vi "Write CFG File.vi"(7 "Section":string, 8 "error in (no error)":errorcluster, 10 "File refnum":T1, 11 "Mag Lab Parameters in":refnum<class "Mag Lab Parameters.lvclass">) -> (0 "error out":errorcluster, 2 "File refnum out":T1, 3 "Mag Lab Parameters out":refnum<class "Mag Lab Parameters.lvclass">)   [LabVIEW 2015, in "Mag Lab Parameters.lvclass"]
uses:
  Mag Lab Parameters.lvclass
  <vilib>/Utility/config.llb/Config Data RefNum.ctl
  <vilib>/Utility/config.llb/NI_LVConfig.lvlib
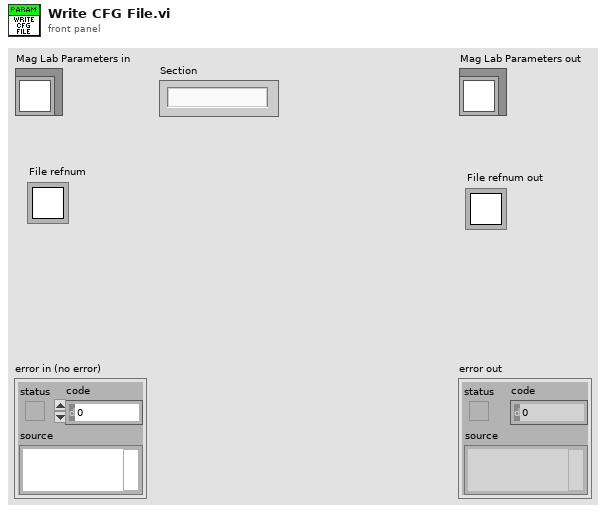
[diagram p1: front panel]
types:
  T1 = typedef "NI_LVConfig.lvlib/Config Data RefNum.ctl" = refnum<k1>
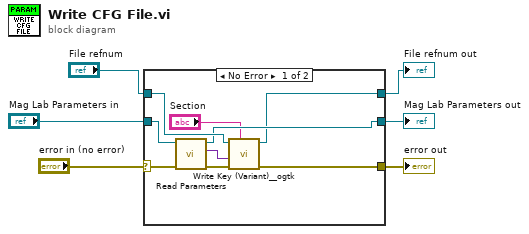
[diagram p0: block diagram]
diagram:
  n1 = case shown="No Error" "error in (no error)" {
    selector: "error in (no error)" -> [w8 w18]
    tunnel: [w9 w18] -> w5
    tunnel: [w13 w17] -> w3
    tunnel: "Mag Lab Parameters in" -> [w15 w17]
    tunnel: "File refnum" -> [w14 w16]
    tunnel: [w10 w16] -> w1
    frame No Error {
      n2 = call-dynamic "Read Parameters.vi"("error in (no error)"=w8, "Mag Lab Parameters in"=w15) -> ("error out"=w7:errorcluster, "Parameters"=w12:variant, "Mag Lab Parameters out"=w13:refnum<class "Mag Lab Parameters.lvclass">)  [unwired: 7 in]
      n3 = call <userlib>:"Write Key (Variant)__ogtk.vi"("section"="Section", "error in (no error)"=w7, "key-value"=w12, "refnum"=w14) -> ("error out"=w9:errorcluster, "refnum out"=w10:T1)  [unwired: 6 in]
    }
    frame Error {
    }
  }
  "error out" <- w5
  "Mag Lab Parameters out" <- w3
  "File refnum out" <- w1
